vi "Host Image Acquisition Module.vi"(8 "error in":errorcluster, 11 "Operation":T3) -> (0 "error out":errorcluster, 1 "Image Acquired":bool, 2 "Acq In Progress":bool, 3 "Image":T2(plugin-control))   [LabVIEW 2013]
uses:
  Host Image Acquisition Module Enum.ctl
  Acquisition Settings Cluster.ctl
  <vilib>/vision/Image Controls.llb/IMAQ Image.ctl
  Image Acquisition Settings FG Enum.ctl
  System Status/Status FG Enum.ctl
  Image Processing/Mask ROI FG Enum.ctl
  <vilib>/rvi/interface/common/niFpgaWaitOnOcc.vi
  <vilib>/FPGAPlugInAG/PCIe-1473R/niLvFpga_Reset_PCIe-1473R.vi
  <vilib>/Utility/error.llb/Error Cluster From Error Code.vi
  <vilib>/rvi/errors/niLvFpgaAdjustHostInterfaceError.vi
  <vilib>/FPGAPlugInAG/PCIe-1473R/niLvFpga_Run_PCIe-1473R.vi
  Globals/Average Sector Data.vi
  <vilib>/FPGAPlugInAG/PCIe-1473R/niLvFpga_Close_PCIe-1473R.vi
  <vilib>/rvi/interface/nirviMethod/nirviMethod.xnode
  FGs/FPGA_Reference.ctl
  FPGA Bitfiles/Simulation_WBA.lvbitx
  <vilib>/rvi/interface/nirviReadWriteControl/nirviReadWriteControl.xnode
  Common/CL Configuration.ctl
  Common/CL Signal Mapping.ctl
  FPGA/Sector/Accumulate/Sector Parameter Cluster.ctl
  <vilib>/rvi/interface/nirviCloseFPGA/nirviCloseFPGA.xnode
  Common/Timing/Timing Lib.lvlib
  NiFpgaLv.dll
  <vilib>/rvi/errors/niLvFpgaMergeErrorWithErrorCode.vi
  <vilib>/FPGAPlugInAG/PCIe-1473R/niLvFpga_ReadFifo_PCIe-1473R.vi
  <vilib>/FPGAPlugInAG/PCIe-1473R/niLvFpga_ConfigureFifo_PCIe-1473R.vi
  <vilib>/FPGAPlugInAG/PCIe-1473R/niLvFpga_StartFifo_PCIe-1473R.vi
panel:
  out "Actual Depth":u32
  out "Target Sim TO":bool
  out "Cam Data Timeout":bool
  out "Sector FIFO Timeout":bool
  out "Host DMA Timeout":bool
  out "Number of Elements to Write Host DMA":u32
  out "Number of Elements to Read Cam Data":u32
  out "Image Data":u64[](array[numeric])
  out "Elements Remaining":u32
  out "Words per image":u32
  out "Num Frames read":u32
  out "DMA Words per Image":u32
  out "Acquire":bool
  in  "Acquisition Settings Cluster":T1={"Image Width"=2040, "Image Height"=1088, "Frames To Acquire"=0, "Signal Mapping"=enum."Basler 10-tap", "DMA Buffer Size\n(In Images)"=64} {"Image Height" max=65535; "Image Width" max=65535 step=40}
  out "Buffer Size":u32
  out "Acq'd Frame Width":u32=2040
  out "DMA Write Timeout":bool
  in  "Start Serial Server":bool
  out "Frames Acq'd":u32=1
  out "Acq'd Frame Height":u32=1088
  out "Initialized":bool
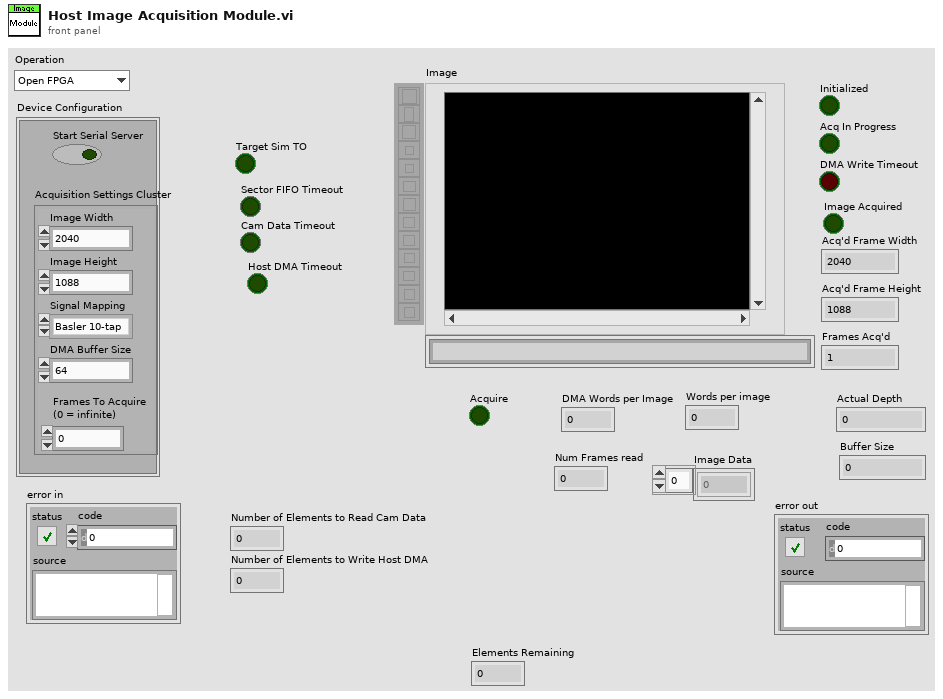
[diagram p1: front panel]
types:
  T1 = typedef "Acquisition Settings Cluster.ctl" = cluster{"Image Width":u32, "Image Height":u32, "Frames To Acquire":u32, "Signal Mapping":enum8{"Standard", "Basler 10-tap", "Vosskühler 10-tap"}, "DMA Buffer Size\n(In Images)":u32}
  T2 = typedef "IMAQ Image.ctl" = refnum<image>
  T3 = typedef "Host Image Acquisition Module Enum.ctl" = enum16{"Open FPGA", "Initialize DMA FIFO", "Load Sim Images", "Initialize Acquisition", "Update Sector Parameters", "Start Acquisition", "Aquire Image", "Read Averages", "Cancel Acquisition", "Close FPGA"}
  T4 = enum8{"Standard", "Basler 10-tap", "Vosskühler 10-tap"}
  T5 = typedef "Image Acquisition Settings FG Enum.ctl" = enum16{"Read", "Write"}
  T6 = typedef "Status FG Enum.ctl" = enum16{"Reset", "Read", "Write"}
  T7 = typedef "Mask ROI FG Enum.ctl" = enum16{"Read", "Write"}
  T8 = enum16{"big-endian, network order", "native, host order", "little-endian"}
  T9 = typedef "FPGA_Reference.ctl" = refnum<k20>
  T10 = typedef "Image Type" = u32
  T11 = typedef "Mask ROI Cluster.ctl" = cluster{"left annulus":T12, "right annulus":T12, "Threshold Range":cluster{"Lower value":dbl, "Upper value":dbl}, "[Avg BG]":u8[], "Number of Sectors":u8, "Left ROI":T13, "Right ROI":T13, "Left Start Angle Duty Cycle":fxp<+,8,0>, "Left End Angle Duty Cycle":fxp<+,8,0>, "Right End Angle Duty Cycle":fxp<+,8,0>, "Right Start Angle Duty Cycle":fxp<+,8,0>, "[Sector ROIs]":T13[]}
  T12 = typedef "IMAQ Circle" = cluster{"Center X":i32, "Center Y":i32, "Inner Radius":i32, "Outer Radius":i32, "Start Angle":dbl, "End Angle":dbl}
  T13 = typedef "ROI Descriptor" = cluster{"Global Rectangle":i32[], "Contours":cluster{"ID":enum32{"External", "Internal"}, "Type":u32, "Coordinates":i32[]}[]}
  T14 = typedef "Sector Parameter Cluster.ctl" = cluster{"Start Angle":fxp<+/-,17,2>, "End Angle":fxp<+/-,17,2>, "Inner Radius":u16, "Outter Radius":u16, "Hinge X":u16, "Hinge Y":u16, "NumWingSectors":u8}
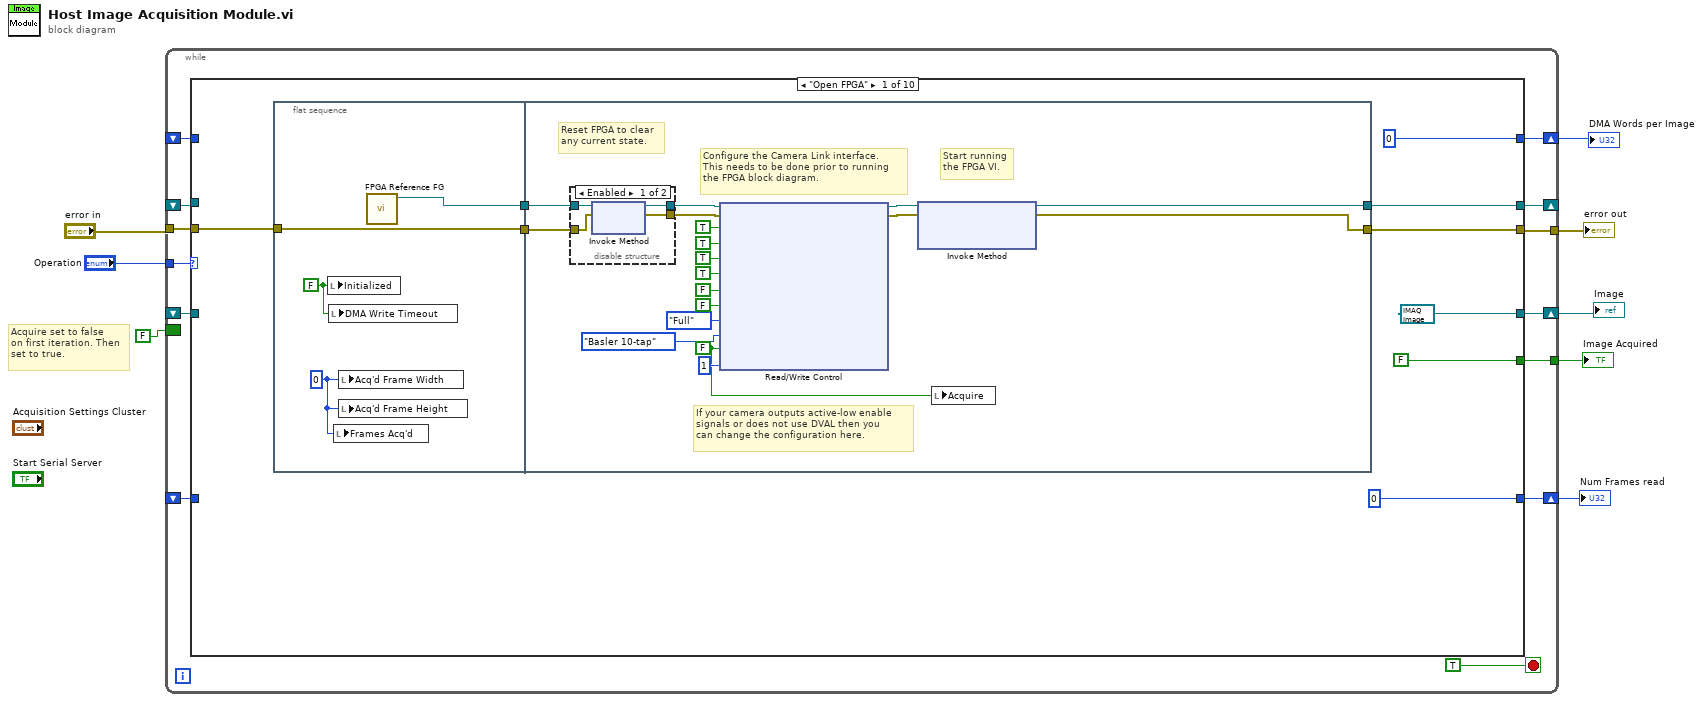
[diagram p0: block diagram]
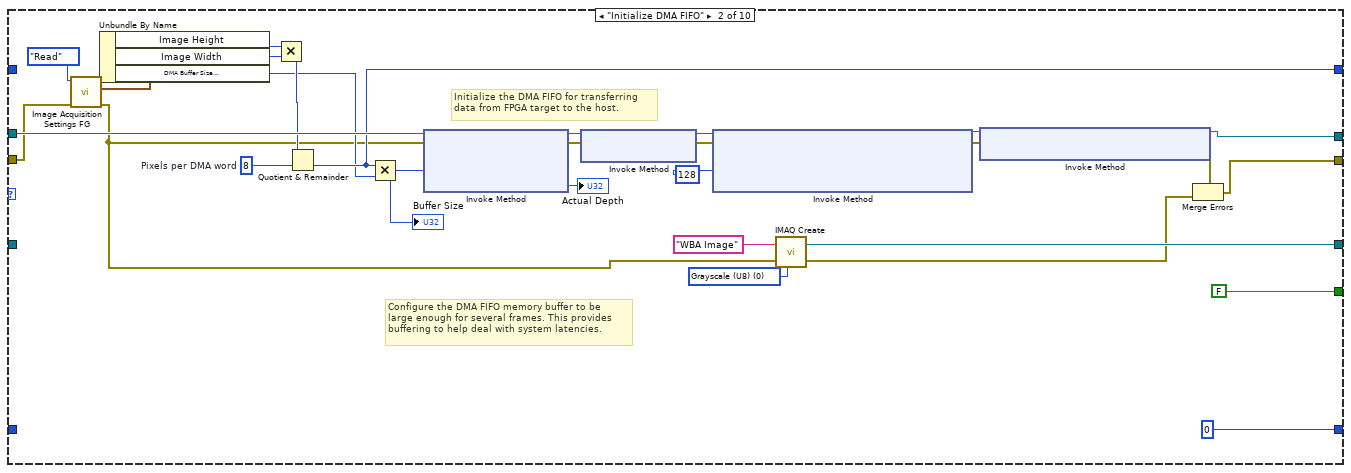
[diagram p3: hidden frame]
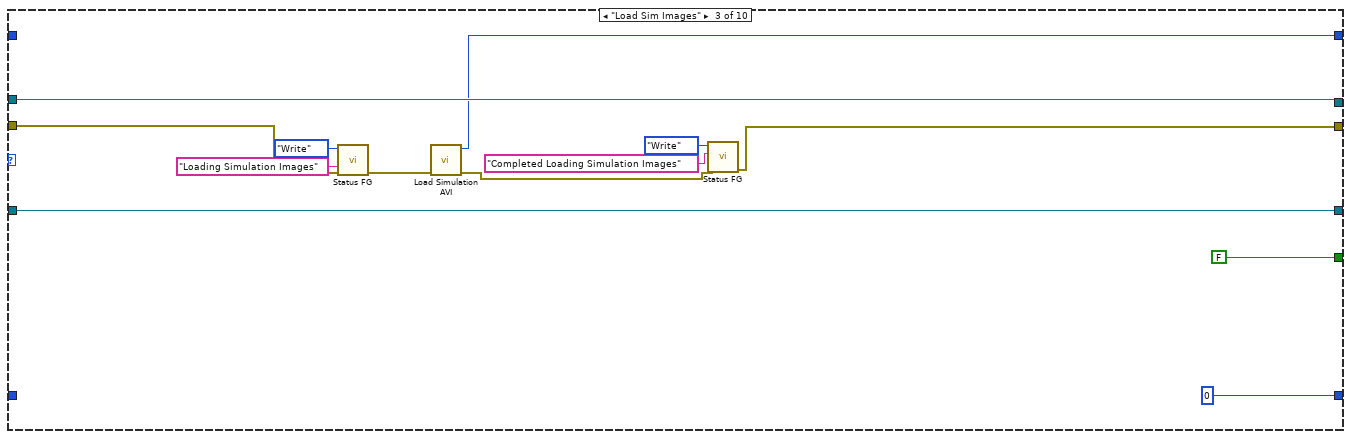
[diagram p4: hidden frame]
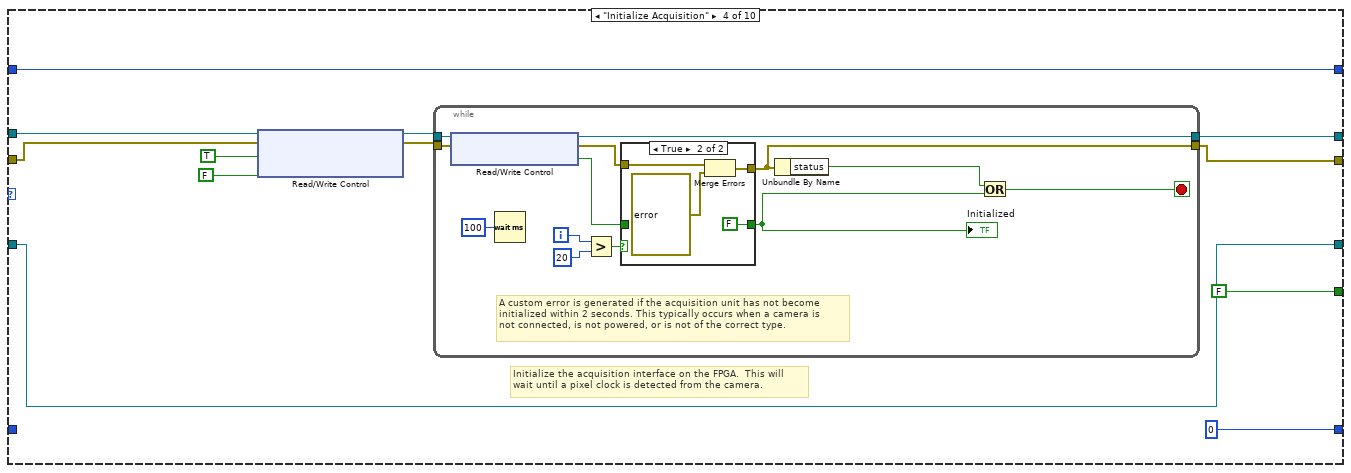
[diagram p5: hidden frame]
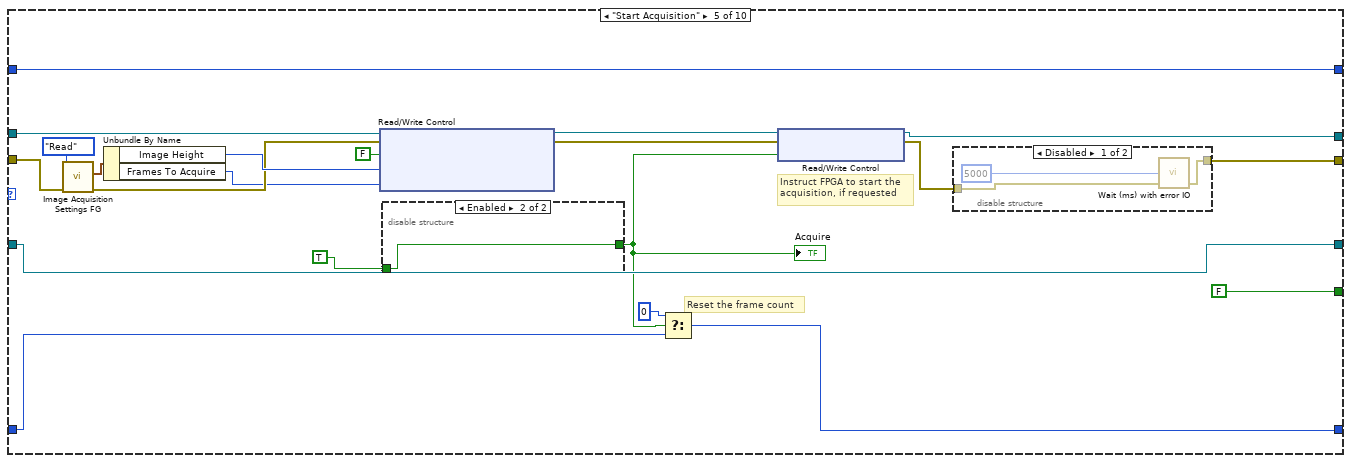
[diagram p7: hidden frame]
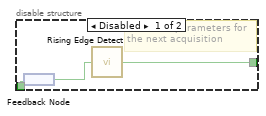
[diagram p9: hidden frame]
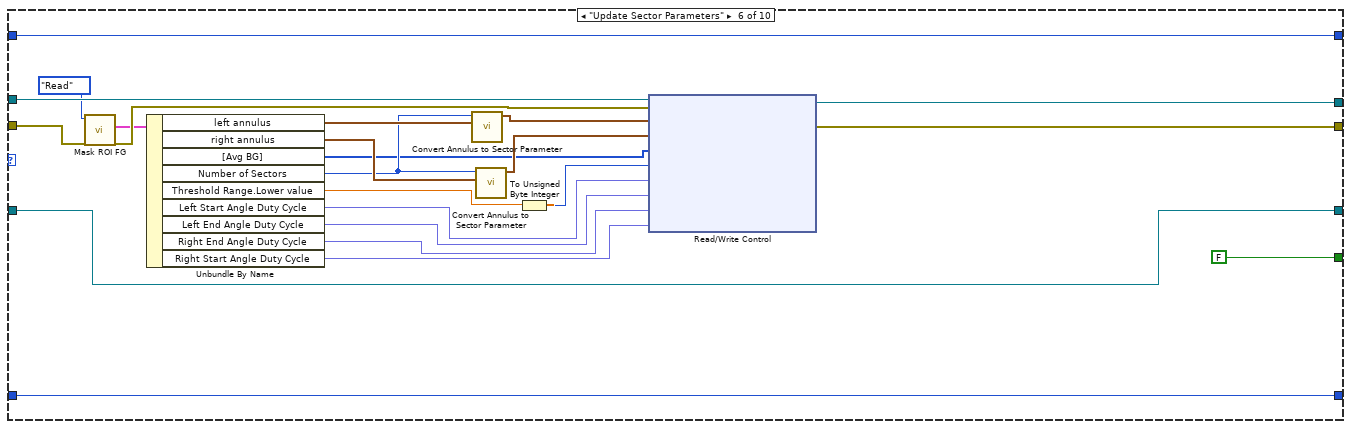
[diagram p10: hidden frame]
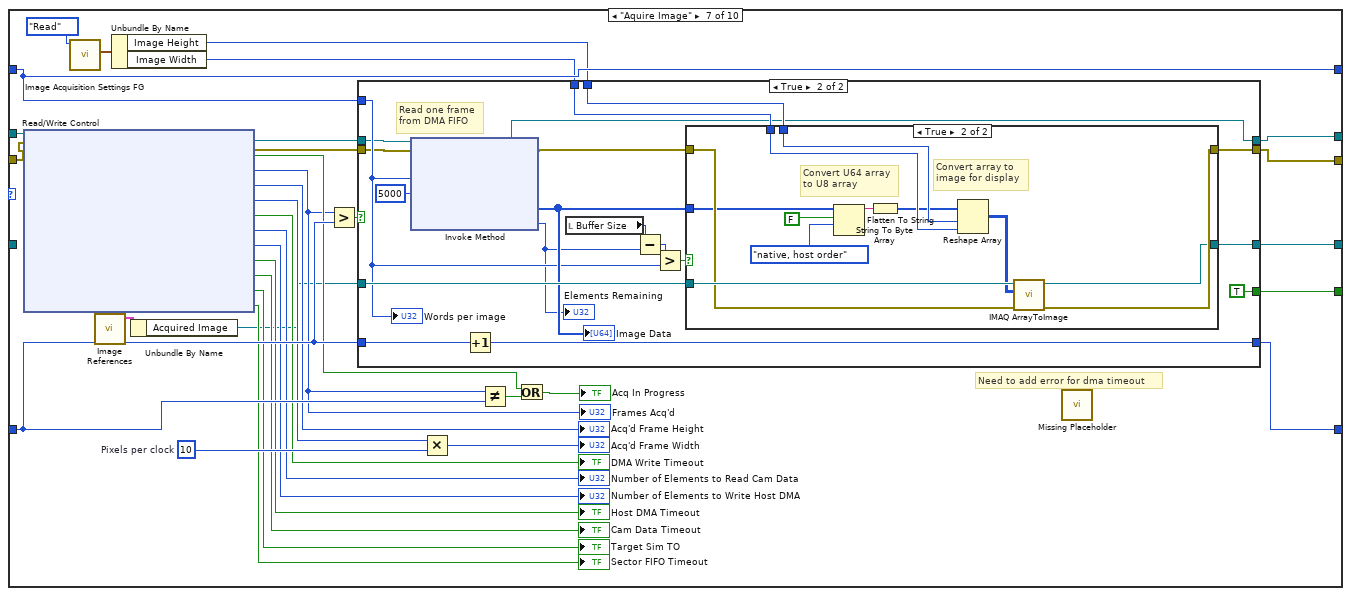
[diagram p11: hidden frame]
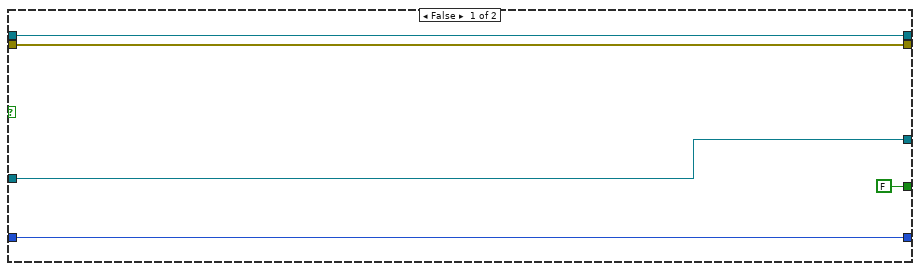
[diagram p12: hidden frame]
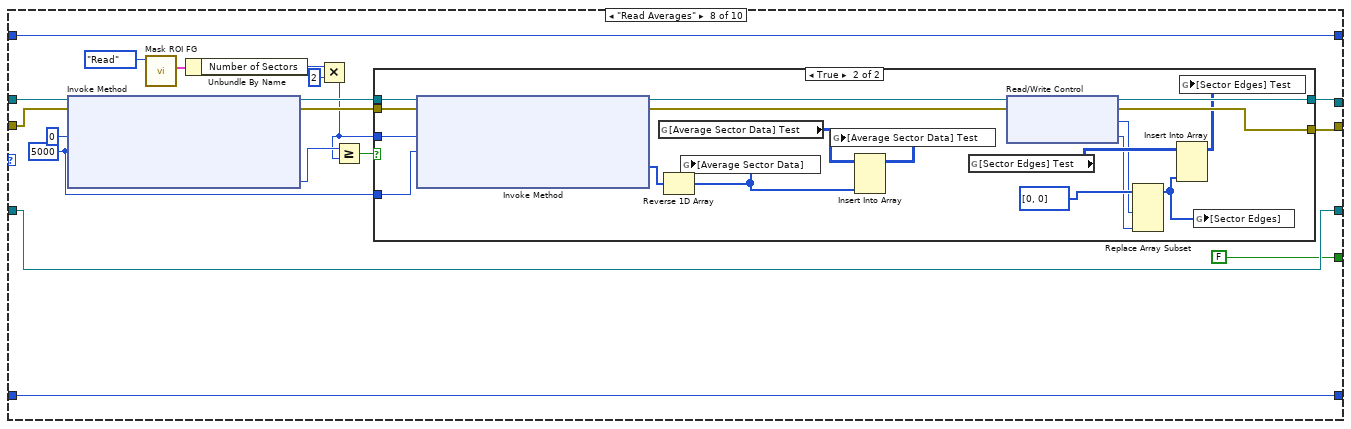
[diagram p14: hidden frame]
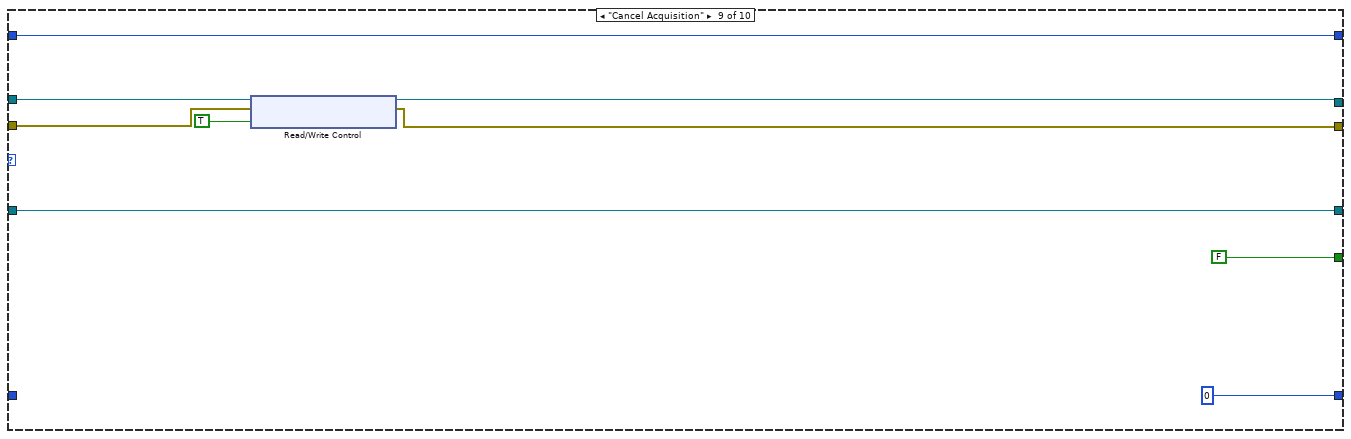
[diagram p16: hidden frame]
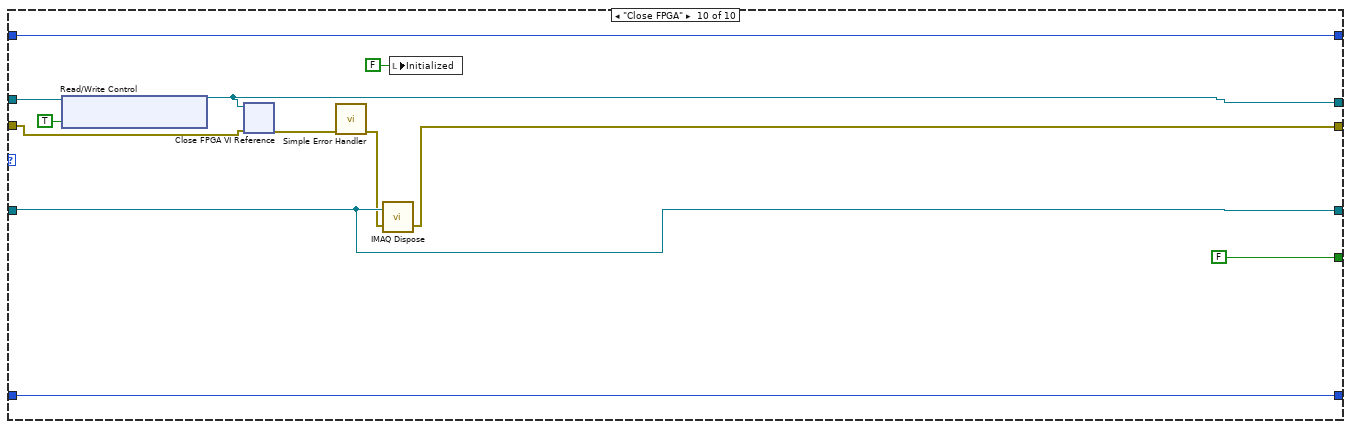
[diagram p17: hidden frame]
diagram:
  # "Acquire set to false\non first iteration. Then\nset to true."
  n1 = while {
    shift-right: [w20] -> _
    shift-left: _ -> [w16]
    tunnel: "error in" -> [w19]
    tunnel: "Operation" -> [w18]
    tunnel: [w17] -> w6
    shift-right: [w15] -> w3
    shift-left: _ -> [w14]
    shift-right: [w13] -> w4
    shift-left: _ -> [w10]
    shift-right: [w12] -> w2
    shift-left: _ -> [w11]
    border: FALSE ("Acquire") -> [_]
    tunnel: [w9] -> w1
    stop <- TRUE stop-if-true
    n2 = case shown="\"Open FPGA\"" w18 {
      tunnel: w19 -> [w30 w83 w95 w106 w151 w181 w210 w266 w299 w308]
      tunnel: [w29 w81 w98 w111 w146 w179 w215 w272 w301 w309] -> w20
      tunnel: [w28 w82 w94 w108 w145 w180 w214 w267 w298 w314] -> w17
      tunnel: w16 -> [_ w87 w98 w112 w152 w183 w216 w273 w302 w310]
      tunnel: [u32 0 w86 w97 w110 w148 w182 w211 w271 w297 w311] -> w15
      tunnel: w14 -> [_ _ _ w110 w148 w182 w211 w271 w297 w311]
      tunnel: [T2 refnum ("New Image") w84 w99 w107 w147 w177 w212 w270 w300 w312] -> w13
      tunnel: [u32 0 u32 0 u32 0 u32 0 w149 w178 w213 w269 u32 0 w313] -> w12
      tunnel: w11 -> [_ _ _ _ w150 w178 w209 w269 _ w313]
      tunnel: w10 -> [_ _ w99 w107 w147 w177 _ w270 w300 w312]
      tunnel: [FALSE ("Image Acquired") FALSE ("Image Acquired") FALSE ("Image Acquired") FALSE ("Image Acquired") FALSE ("Image Acquired") FALSE ("Image Acquired") w208 FALSE ("Image Acquired") FALSE ("Image Acquired") FALSE ("Image Acquired")] -> w9
      frame "Open FPGA" {
        n3 = flat-sequence {
          tunnel: w30 -> [w31]
          tunnel: [w32] -> w27
          tunnel: [w31] -> w26
          tunnel: [w49] -> w28
          tunnel: [w50] -> w29
          tunnel: w27 -> [w52]
          tunnel: w26 -> [w51]
          frame #0 {
            w33 = u32 0 ("Acq'd Frame Width")
            w34 = FALSE ("Initialized")
            n4 = local write "Initialized"(w34) -> ()
            n5 = local write "DMA Write Timeout"(w34) -> ()
            n6 = local write "Frames Acq'd"(w33) -> ()
            n7 = local write "Acq'd Frame Width"(w33) -> ()
            n8 = local write "Acq'd Frame Height"(w33) -> ()
            n9 = call "FPGA Reference FG.vi"() -> ("FPGA VI Reference Out"=w32:T9)  [unwired: 11 in]
          }
          frame #1 {
            w35 = FALSE ("Acq Control.Acquire")
            # "If your camera outputs active-low enable\nsignals or does not use DVAL then you \ncan change the configuration here."
            # "Start running\nthe FPGA VI."
            # "Reset FPGA to clear\nany current state."
            # "Configure the Camera Link interface.\nThis needs to be done prior to running\nthe FPGA block diagram."
            n10 = disable-structure shown="Enabled" {
              disable-tunnel: [w56 w58] -> w42
              disable-tunnel: [w55 w57] -> w40
              disable-tunnel: w52 -> [w54 w58]
              disable-tunnel: w51 -> [w53 w57]
              frame Enabled {
                n11 = xnode "Invoke Method"("FPGA VI Reference In"=w54, "error in"=w53) -> ("FPGA VI Reference Out"=w56:T9, "error out"=w55:errorcluster)
              }
              frame Disabled {
              }
            }
            n12 = xnode "Read/Write Control"("FPGA VI Reference In"=w42, "error in"=w40, "CL Config.FVAL Active High"=TRUE ("IO Module Config.CL FVAL Active High"), "CL Config.LVAL Active High"=TRUE ("IO Module Config.CL LVAL Active High"), "CL Config.DVAL Active High"=TRUE ("IO Module Config.CL DVAL Active High"), "CL Config.Spare Active High"=TRUE ("IO Module Config.CL Spare Active High"), "CL Config.Line Scan"=FALSE, "Acq Control.Ignore DVAL"=FALSE ("CL Config.Line Scan"), "CL Config.Configuration"=enum8{"Base", "Medium", "Full"}."Full", "CL Config.Signal Mapping"=T4."Basler 10-tap", "Acq Control.Acquire"=w35, "# of Frames to Average"=u8 1) -> ("FPGA VI Reference Out"=w39:T9, "error out"=w41:errorcluster)
            n13 = xnode "Invoke Method"("FPGA VI Reference In"=w39, "error in"=w41) -> ("FPGA VI Reference Out"=w50:T9, "error out"=w49:errorcluster)  [unwired: 1 in]
            n14 = local write "Acquire"(w35) -> ()
          }
        }
      }
      frame "Initialize DMA FIFO" {
        w73 = T10 0 items=["Grayscale (U8)", "Grayscale (I16)", "Grayscale (SGL)", "Complex (CSG)", "RGB (U32)", "HSL (U32)", "RGB (U64)", "Grayscale (U16)"] ("Image Type")
        w76 = u32 8  # Pixels per DMA word
        # "Configure the DMA FIFO memory buffer to be\nlarge enough for several frames. This provides\nbuffering to help deal with system latencies."
        # "Initialize the DMA FIFO for transferring\ndata from FPGA target to the host."
        n15 = call "Image Acquisition Settings FG.vi"("error in (no error)"=w83, "Operation"=Image_Acquisition_Settings_FG_Enum."Read") -> ("error out"=w66:errorcluster, "Acquisition Settings Out"=w71:T1)  [unwired: 8 in]
        n16 = Unbundle By Name(w71) -> ("Image Height"=w70:u32, "Image Width"=w69:u32, "DMA Buffer Size\n(In Images)"=w68:u32)
        n17 = Multiply(x=w70, y=w69) -> (x*y=w75:u32)
        n18 = Quotient & Remainder(x=w75, y=w76) -> (floor(x/y)=w86:u32)  [unwired: 1 out]
        n19 = Multiply(x=w86, y=w68) -> (x*y=w77:u32)
        "Buffer Size" <- w77
        n20 = xnode "Invoke Method"("FPGA VI Reference In"=w87, "error in"=w66, "Requested Depth"=w77) -> ("FPGA VI Reference Out"=w79:T9, "error out"=w78:errorcluster, "Actual Depth"=→"Actual Depth":u32)
        n21 = xnode "Invoke Method"("FPGA VI Reference In"=w79, "error in"=w78) -> ("FPGA VI Reference Out"=w64:T9, "error out"=w62:errorcluster)
        n22 = xnode "Invoke Method"("FPGA VI Reference In"=w64, "error in"=w62, "Requested Depth"=u32 128) -> ("FPGA VI Reference Out"=w61:T9, "error out"=w60:errorcluster)  [unwired: 1 out]
        n23 = call "IMAQ Create"("Image Name"="WBA Image", "Image Type"=w73, "error in (no error)"=w66) -> ("New Image"=w84:T2, "error out"=w65:errorcluster)  [unwired: 2 in]
        n24 = xnode "Invoke Method"("FPGA VI Reference In"=w61, "error in"=w60) -> ("FPGA VI Reference Out"=w81:T9, "error out"=w59:errorcluster)
        n25 = Merge Errors(w59, w65) -> (w82:errorcluster)
      }
      frame "Load Sim Images" {
        n26 = call "Status FG.vi"("error in (no error)"=w95, "Status In"="Loading Simulation Images", "Operation"=Status_FG_Enum."Write") -> ("error out"=w93:errorcluster)  [unwired: 7 in, 1 out]
        n27 = call "Load Simulation AVI.vi"("error in (no error)"=w93) -> ("error out"=w89:errorcluster, "Words per image"=w97:u32)  [unwired: 9 in]
        n28 = call "Status FG.vi"("error in (no error)"=w89, "Status In"="Completed Loading Simulation Images", "Operation"=Status_FG_Enum."Write") -> ("error out"=w94:errorcluster)  [unwired: 7 in, 1 out]
      }
      frame "Initialize Acquisition" {
        # "Initialize the acquisition interface on the FPGA.  This will\nwait until a pixel clock is detected from the camera."
        n29 = xnode "Read/Write Control"("FPGA VI Reference In"=w112, "error in"=w106, "Acq Control.Initialize"=TRUE ("Arm Acquisition"), "Acq Control.Cancel Acq"=FALSE) -> ("FPGA VI Reference Out"=w104:T9, "error out"=w103:errorcluster)
        n30 = while {
          tunnel: w104 -> [w121]
          tunnel: w103 -> [w120]
          tunnel: [w119] -> w111
          tunnel: [w122] -> w108
          i -> [w115]
          stop <- w125 stop-if-true
          # "A custom error is generated if the acquisition unit has not become\ninitialized within 2 seconds. This typically occurs when a camera is\nnot connected, is not powered, or is not of the correct type."
          n31 = xnode "Read/Write Control"("FPGA VI Reference In"=w121, "error in"=w120) -> ("FPGA VI Reference Out"=w119:T9, "error out"=w118:errorcluster, "Acq Status.Initialized"=w117:bool)
          n32 = Wait (ms)(milliseconds to wait=u32 100) -> ()  [unwired: 1 out]
          n33 = Greater?(x=w115, y=20) -> (0:w116:bool)
          n34 = case shown="True" w116 {
            tunnel: [w127 FALSE] -> w113
            tunnel: w117 -> [w127 _]
            tunnel: w118 -> [w126 w129]
            tunnel: [w126 w131] -> w122
            frame False {
            }
            frame True {
              n35 = Merge Errors(w129, errorcluster {"status"=TRUE, "code"=-8999, "source"="Acquisition Initialization: This error typically occurs when a camera is not properly connected, is not powered, or is not of the correct type."} ("error in")) -> (w131:errorcluster)
            }
          }
          "Initialized" <- w113
          n36 = Unbundle By Name(w122) -> ("status"=w124:bool)
          n37 = Or(x=w124, y=w113) -> (x .or. y?=w125:bool)
        }
      }
      frame "Start Acquisition" {
        # "Reset the frame count"
        # "Instruct FPGA to start the\nacquisition, if requested"
        n38 = call "Image Acquisition Settings FG.vi"("error in (no error)"=w151, "Operation"=Image_Acquisition_Settings_FG_Enum."Read") -> ("error out"=w137:errorcluster, "Acquisition Settings Out"=w143:T1)  [unwired: 8 in]
        n39 = Unbundle By Name(w143) -> ("Image Height"=w138:u32, "Frames To Acquire"=w134:u32)
        n40 = xnode "Read/Write Control"("FPGA VI Reference In"=w152, "error in"=w137, "Acq Control.Cancel Acq"=FALSE, "Acq Control.Line Scan Height"=w138, "Acq Control.Frames To Acq"=w134) -> ("FPGA VI Reference Out"=w132:T9, "error out"=w133:errorcluster)
        n41 = disable-structure shown="Enabled" {
          disable-tunnel: [w159 w160] -> w140
          disable-tunnel: TRUE ("Acquire") -> [w157 w160]
          frame Disabled {
            # "Write the parameters for\nthe next acquisition"
            n42 = feedback #1() -> (w158:bool)
            n43 = feedback-in #1(w157) -> ()
            n44 = call "Rising Edge Detect.vi"("Input"=w158) -> ("Pulse"=w159:bool)  [unwired: 4 in]
          }
          frame Enabled {
          }
        }
        "Acquire" <- w140
        n45 = Select(t=u32 0, s=w140, f=w150) -> (s? t:f=w149:u32)
        n46 = xnode "Read/Write Control"("FPGA VI Reference In"=w132, "error in"=w133, "Acq Control.Acquire"=w140) -> ("FPGA VI Reference Out"=w146:T9, "error out"=w135:errorcluster)
        n47 = disable-structure shown="Disabled" {
          disable-tunnel: w135 -> [w154 w156]
          disable-tunnel: [w153 w156] -> w145
          frame Disabled {
            n48 = call "Wait (ms) with error IO.vi"("error in (no error)"=w154, "milliseconds to wait"=u32 5000) -> ("error out"=w153:errorcluster)  [unwired: 3 in]
          }
          frame Enabled {
          }
        }
      }
      frame "Update Sector Parameters" {
        n49 = call "Mask ROI FG.vi"("error in (no error)"=w181, "Operation"=Mask_ROI_FG_Enum."Read") -> ("error out"=w175:errorcluster, "Mask ROI Out"=w173:T11)  [unwired: 8 in]
        n50 = Unbundle By Name(w173) -> ("left annulus"=w172:T12, "right annulus"=w170:T12, "[Avg BG]"=w167:u8[], "Number of Sectors"=w169:u8, "Threshold Range.Lower value"=w166:dbl, "Left Start Angle Duty Cycle"=w164:fxp<+,8,0>, "Left End Angle Duty Cycle"=w163:fxp<+,8,0>, "Right End Angle Duty Cycle"=w162:fxp<+,8,0>, "Right Start Angle Duty Cycle"=w161:fxp<+,8,0>)
        n51 = call "Convert Annulus to Sector Parameter.vi"("Annulus"=w172, "NumWingSectors"=w169) -> ("Sector Parameter"=w171:T14)  [unwired: 9 in]
        n52 = call "Convert Annulus to Sector Parameter.vi"("Annulus"=w170, "NumWingSectors"=w169) -> ("Sector Parameter"=w168:T14)  [unwired: 9 in]
        n53 = To Unsigned Byte Integer(number=w166) -> (unsigned 8bit integer=w165:u8)
        n54 = xnode "Read/Write Control"("FPGA VI Reference In"=w183, "error in"=w175, "Sector Parameters Left"=w171, "Sector Parameters Right"=w168, "[Average BG Intensity]"=w167, "Sector Threshold"=w165, "Left Start Angle Duty Cycle"=w164, "Left End Angle Duty Cycle"=w163, "Right End Angle Duty Cycle"=w162, "Right Start Angle Duty Cycle"=w161) -> ("FPGA VI Reference Out"=w179:T9, "error out"=w180:errorcluster)
      }
      frame "Aquire Image" {
        w203 = u32 10  # Pixels per clock
        # "Need to add error for dma timeout"
        n55 = xnode "Read/Write Control"("FPGA VI Reference In"=w216, "error in"=w210) -> ("FPGA VI Reference Out"=w207:T9, "error out"=w206:errorcluster, "Acq Status.Acq In Progress"=w195:bool, "Acq Status.Frames Acq'd"=w194:u32, "Acq Status.Lines Per Frame"=→"Acq'd Frame Height":u32, "Acq Status.Clocks Per Line"=w202:u32, "Acq Status.DMA Write Timeout"=→"DMA Write Timeout":bool, "Number of Elements to Read Cam Data"=→"Number of Elements to Read Cam Data":u32, "Number of Elements to Write Host DMA"=→"Number of Elements to Write Host DMA":u32, "Host DMA Timeout"=→"Host DMA Timeout":bool, "Cam Data Timeout"=→"Cam Data Timeout":bool, "Target Sim TO"=→"Target Sim TO":bool, "Sector FIFO Timeout"=→"Sector FIFO Timeout":bool)
        "Frames Acq'd" <- w194
        n56 = call "Image Acquisition Settings FG.vi"("Operation"=Image_Acquisition_Settings_FG_Enum."Read") -> ("Acquisition Settings Out"=w198:T1)  [unwired: 9 in, 1 out]
        n57 = call "Image References.vi"() -> ("Images"=w185:cluster{"Acquired Image":T2, "Display Image":T2})  [unwired: 10 in, 1 out]
        n58 = Unbundle By Name(w198) -> ("Image Height"=w197:u32, "Image Width"=w196:u32)
        n59 = Unbundle By Name(w185) -> ("Acquired Image"=w184:T2)
        n60 = Greater?(x=w194, y=w209) -> (0:w205:bool)
        n61 = case shown="True" w205 {
          tunnel: w207 -> [w220 w223]
          tunnel: w206 -> [w219 w224]
          tunnel: w197 -> [_ w240]
          tunnel: w196 -> [_ w239]
          tunnel: w184 -> [w221 w238]
          tunnel: [w219 w236] -> w214
          tunnel: [w220 w235] -> w215
          tunnel: w209 -> [w218 w234]
          tunnel: [w218 w233] -> w213
          tunnel: w211 -> [_ w230]
          tunnel: [w221 w229] -> w212
          tunnel: [FALSE ("Image Acquired") TRUE ("Image Acquired")] -> w208
          frame False {
          }
          frame True {
            # "Read one frame\nfrom DMA FIFO"
            n62 = xnode "Invoke Method"("FPGA VI Reference In"=w223, "error in"=w224, "Number of Elements"=w230, "Timeout (ms)"=5000) -> ("FPGA VI Reference Out"=w235:T9, "error out"=w237:errorcluster, "Data"=w232:u64[], "Elements Remaining"=w227:u32)
            "Elements Remaining" <- w227
            "Image Data" <- w232
            n63 = Increment(x=w234) -> (x+1=w233:u32)
            n64 = local read "Buffer Size"() -> (w228:u32)
            n65 = Subtract(x=w228, y=w227) -> (x-y=w226:u32)
            n66 = Greater?(x=w226, y=w230) -> (0:w231:bool)
            n67 = case shown="True" w231 {
              tunnel: w240 -> [_ w254]
              tunnel: w239 -> [_ w253]
              tunnel: w238 -> [w241 w252]
              tunnel: w237 -> [w242 w251]
              tunnel: [w242 w250] -> w236
              tunnel: w232 -> [_ w247]
              tunnel: [w241 w243] -> w229
              frame False {
                # "Do not display the image if we're\nfalling behind in the acquisition."
              }
              frame True {
                # "Convert U64 array\nto U8 array"
                # "Convert array to\nimage for display"
                n68 = Flatten To String(anything=w247, prepend array or string size? (T)=FALSE, byte order (0:big-endian, network order)=T8."native, host order") -> (data string=w245:string)  [unwired: 1 in, 2 out]
                n69 = String To Byte Array(string=w245) -> (unsigned byte array=w244:u8[])
                n70 = Reshape Array(w244, w254, w253) -> (w249:u8[][])
                n71 = call "IMAQ ArrayToImage"("error in (no error)"=w251, "Image Pixels (U8)"=w249, "Image"=w252) -> ("error out"=w250:errorcluster, "Image Out"=w243:T2)  [unwired: 7 in]
              }
            }
            "Words per image" <- w230
          }
        }
        n72 = Multiply(x=w202, y=w203) -> (x*y=→"Acq'd Frame Width":u32)
        n73 = Not Equal?(x=w194, y=w209) -> (x != y?=w193:bool)
        n74 = Or(x=w195, y=w193) -> (x .or. y?=→"Acq In Progress":bool)
        n75 = call "Missing Placeholder.vi"() -> ()  [unwired: 12 in]
      }
      frame "Read Averages" {
        w262 = 5000 ("Timeout (ms)")
        n76 = xnode "Invoke Method"("FPGA VI Reference In"=w273, "error in"=w266, "Number of Elements"=u32 0, "Timeout (ms)"=w262) -> ("FPGA VI Reference Out"=w264:T9, "error out"=w263:errorcluster, "Elements Remaining"=w257:u32)  [unwired: 1 out]
        n77 = call "Mask ROI FG.vi"("Operation"=Mask_ROI_FG_Enum."Read") -> ("Mask ROI Out"=w260:T11)  [unwired: 9 in, 1 out]
        n78 = Unbundle By Name(w260) -> ("Number of Sectors"=w258:u8)
        n79 = Multiply(x=w258, y=u8 2) -> (x*y=w256:u8)
        n80 = Greater Or Equal?(x=w257, y=w256) -> (x >= y?=w259:bool)
        n81 = case shown="True" w259 {
          tunnel: w264 -> [w275 w293]
          tunnel: w263 -> [w274 w292]
          tunnel: w262 -> [_ w291]
          tunnel: [w275 w284] -> w272
          tunnel: [w274 w285] -> w267
          tunnel: w256 -> [_ w290]
          frame False {
          }
          frame True {
            n82 = xnode "Invoke Method"("FPGA VI Reference In"=w293, "error in"=w292, "Number of Elements"=w290, "Timeout (ms)"=w291) -> ("FPGA VI Reference Out"=w287:T9, "error out"=w286:errorcluster, "Data"=w281:u8[])  [unwired: 1 out]
            n83 = global read "Average Sector Data.vi" "[Average Sector Data] Test"() -> (w289:u8[][])
            n84 = Reverse 1D Array(array=w281) -> (reversed array=w280:u8[])
            n85 = global write "Average Sector Data.vi" "[Average Sector Data]"(w280) -> ()
            n86 = Insert Into Array(array=w289, new element=w280) -> (w288:u8[][])  [unwired: 2 in]
            n87 = global write "Average Sector Data.vi" "[Average Sector Data] Test"(w288) -> ()
            n88 = global read "Average Sector Data.vi" "[Sector Edges] Test"() -> (w283:u8[][])
            n89 = xnode "Read/Write Control"("FPGA VI Reference In"=w287, "error in"=w286) -> ("FPGA VI Reference Out"=w284:T9, "error out"=w285:errorcluster, "Right Sector Edge"=w278:u8, "Left Sector Edge"=w277:u8)
            n90 = Replace Array Subset(array=u8[] [0, 0] ("[Sector Edges]"), new element #1=w278, new element #2=w277) -> (w276:u8[])  [unwired: 2 in]
            n91 = Insert Into Array(array=w283, new element=w276) -> (w282:u8[][])  [unwired: 2 in]
            n92 = global write "Average Sector Data.vi" "[Sector Edges] Test"(w282) -> ()
            n93 = global write "Average Sector Data.vi" "[Sector Edges]"(w276) -> ()
          }
        }
      }
      frame "Cancel Acquisition" {
        n94 = xnode "Read/Write Control"("FPGA VI Reference In"=w302, "error in"=w299, "Acq Control.Cancel Acq"=TRUE) -> ("FPGA VI Reference Out"=w301:T9, "error out"=w298:errorcluster)
      }
      frame "Close FPGA" {
        n95 = xnode "Read/Write Control"("FPGA VI Reference In"=w310, "Acq Control.Cancel Acq"=TRUE) -> ("FPGA VI Reference Out"=w309:T9)  [unwired: 1 in, 1 out]
        n96 = xnode "Close FPGA VI Reference"("FPGA VI Reference In"=w309, "error in"=w308) -> ("error out"=w306:errorcluster)
        n97 = call <vilib>:"Simple Error Handler.vi"("error in (no error)"=w306) -> ("error out"=w304:errorcluster)  [unwired: 4 in, 4 out]
        n98 = call "IMAQ Dispose"("Image"=w312, "error in (no error)"=w304) -> ("error out"=w314:errorcluster)  [unwired: 4 in]
        n99 = local write "Initialized"(FALSE ("Initialized")) -> ()
      }
    }
  }
  "error out" <- w6
  "Image" <- w4
  "DMA Words per Image" <- w3
  "Num Frames read" <- w2
  "Image Acquired" <- w1
